vi "FPGA Wait On IRQ.vi"(6 "Timeout (ms)":u32=5000, 8 "error in (no error)":errorcluster, 10 "IRQ":u32, 11 "FPGA Session In":refnum<class "FPGA Interface Base.lvclass">) -> (0 "error out":errorcluster, 2 "IRQ Asserted":u32, 3 "FPGA Session Out":refnum<class "FPGA Interface Base.lvclass">, 4 "Timed Out?":bool)   [LabVIEW 2010, in "FPGA Interface Base.lvclass"]
uses:
  <userlib>/_FPGA Interface Advanced Tools/FPGA Interface Base/FPGA Interface Base.lvclass
  <userlib>/_FPGA Interface Advanced Tools/FPGA Interface Base/Accessors/FPGA Read Session.vi
  <userlib>/_FPGA Interface Advanced Tools/FPGA Interface Base/Accessors/FPGA Read IRQ Context Queue.vi
  <vilib>/Utility/error.llb/Error Cluster From Error Code.vi
  <userlib>/_FPGA Interface Advanced Tools/FPGA Interface Wrapper/FPGA Interface Wrapper.lvlib
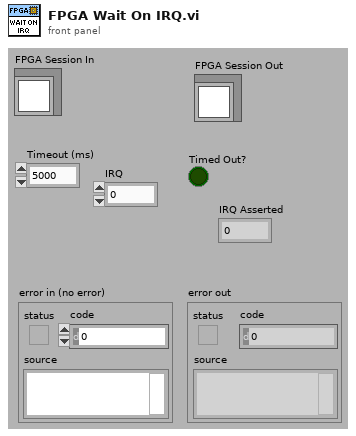
[diagram p1: front panel]
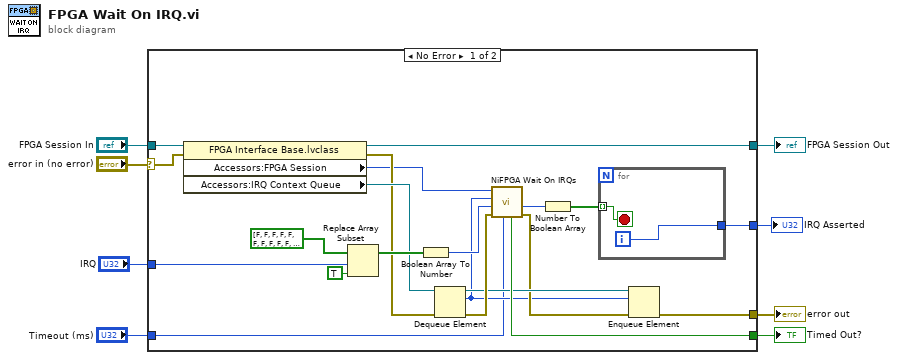
[diagram p0: block diagram]
diagram:
  n1 = case shown="No Error" "error in (no error)" {
    selector: "error in (no error)" -> [w12 w33]
    tunnel: [w17 w33] -> w4
    tunnel: [w13 w32] -> w7
    tunnel: "FPGA Session In" -> [w14 w32]
    tunnel: "IRQ" -> [w24 _]
    tunnel: [w21 _] -> w1
    tunnel: [w28 _] -> w5
    tunnel: "Timeout (ms)" -> [w15 _]
    frame No Error {
      n2 = property class="FPGA Interface Base.lvclass"(reference=w14, error in=w12) -> (reference out=w13:refnum<class "FPGA Interface Base.lvclass">, error out=w10:errorcluster, "Accessors:FPGA Session"=w9:u32, "Accessors:IRQ Context Queue"=w11:refnum<queue>)
      n3 = Replace Array Subset(array=bool[] [FALSE, FALSE, FALSE, FALSE, FALSE, FALSE, FALSE, FALSE, FALSE, FALSE, FALSE, FALSE, FALSE, FALSE, FALSE, FALSE, FALSE, FALSE, FALSE, FALSE, FALSE, FALSE, FALSE, FALSE, FALSE, FALSE, FALSE, FALSE, FALSE, FALSE, FALSE, FALSE], new element=TRUE ("new element/subarray"), index=w24) -> (w26:bool[])
      n4 = Boolean Array To Number(Boolean array=w26) -> (number=w23:u32)
      n5 = Dequeue Element(queue=w11, error in (no error)=w10) -> (queue out=w20:refnum<queue>, element=w18:u32, error out=w27:errorcluster)  [unwired: 1 in, 1 out]
      n6 = call <userlib>:"NiFPGA Wait On IRQs.vi"("Timeout"=w15, "error in (no error)"=w27, "IRQs"=w23, "Context"=w18, "Session In"=w9) -> ("error out"=w19:errorcluster, "IRQs Asserted"=w29:u32, "Timed Out?"=w28:bool)  [unwired: 3 in, 1 out]
      n7 = Number To Boolean Array(number=w29) -> (Boolean array=w22:bool[])
      n8 = for {
        tunnel: w22 -> [w30] mode=indexing
        tunnel: [w31] -> w21
        i -> [w31]
        stop <- w30 stop-if-true
      }
      n9 = Enqueue Element(queue=w20, element=w18, error in (no error)=w19) -> (error out=w17:errorcluster)  [unwired: 1 in, 2 out]
    }
    frame Error {
    }
  }
  "error out" <- w4
  "Timed Out?" <- w5
  "FPGA Session Out" <- w7
  "IRQ Asserted" <- w1
